vi "CreateSequence_Main.vi"(0 "Project Path":path, 5 "Measurement Name":string, 11 "error in (no error)":errorcluster) -> (15 "Error Out":errorcluster)   [LabVIEW 2021, in "Create Sequence.lvlib"]
uses:
  Create Sequence.lvlib
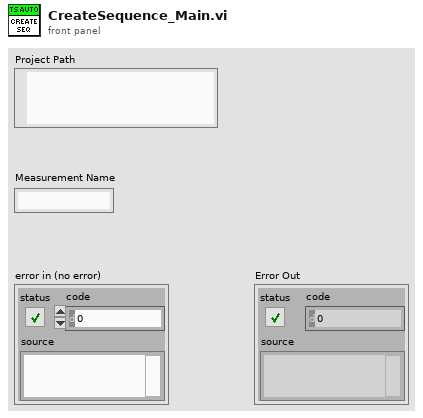
[diagram p1: front panel]
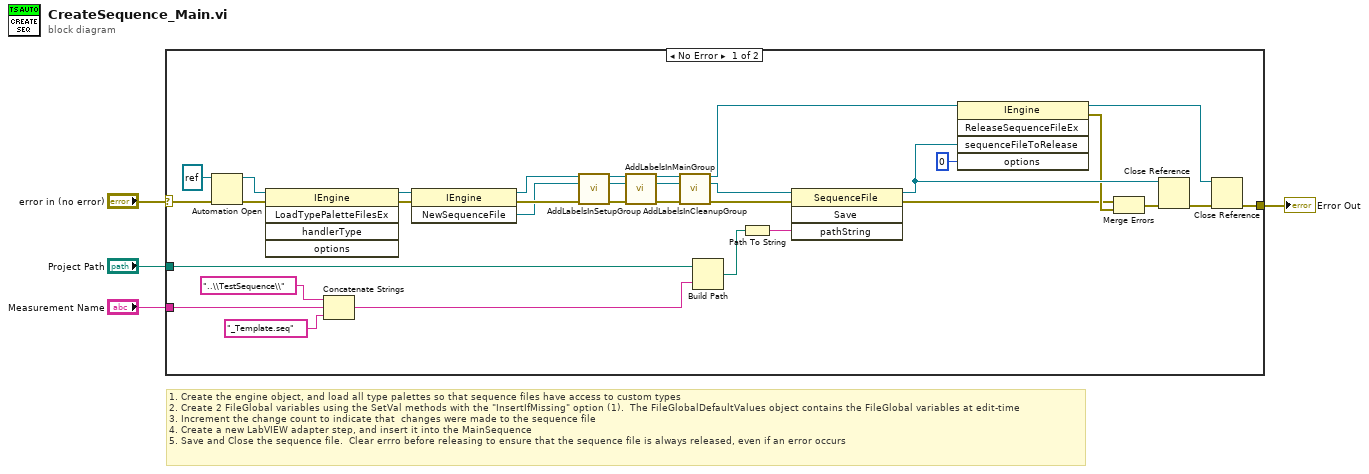
[diagram p0: block diagram]
diagram:
  # "1. Create the engine object, and load all type palettes so that sequence files have access to custom types\n2. Create 2 FileGlobal variables using the SetVal methods with the \"InsertIfMissing\" option (1).  The FileGlobalDefaultValues object contains the FileGlobal variables at edit-time\n3. Increment the change count to indicate that  changes were made to the sequence file\n4. Create a new LabVIEW adapter step, and insert it into the MainSequence\n5. Save and Close the sequence file.  Clear errro before releasing to ensure that the sequence file is always released, even if an error occurs"
  n1 = case shown="No Error" "error in (no error)" {
    selector: "error in (no error)" -> [w17 w38]
    tunnel: [w29 w38] -> w4
    tunnel: "Measurement Name" -> [w15 _]
    tunnel: "Project Path" -> [w5 _]
    frame No Error {
      n2 = Automation Open(error in (no error)=w17, Automation Refnum=refnum<k7> refnum) -> (Automation Refnum=w21:refnum<k7>, error out=w25:errorcluster)  [unwired: 2 in]
      n3 = invoke class="IEngine" method="LoadTypePaletteFilesEx"(reference=w21, error in=w25) -> (reference out=w26:refnum<k7>, error out=w24:errorcluster)  [unwired: 3 in, 3 out]
      n4 = Concatenate Strings("..\\TestSequence\\" ("string"), w15, "_Template.seq" ("string")) -> (w13:string)
      n5 = invoke class="IEngine" method="NewSequenceFile"(reference=w26, error in=w24) -> (reference out=w28:refnum<k7>, error out=w27:errorcluster, "NewSequenceFile"=w22:refnum<k7>)  [unwired: 1 in]
      n6 = call "AddLabelsInSetupGroup.vi"("Engine In"=w28, "SequenceFile In"=w22, "Error In"=w27) -> ("Engine Out"=w11:refnum<k7>, "SequenceFile Out"=w9:refnum<k7>, "Error Out"=w7:errorcluster)  [unwired: 10 in]
      n7 = call "AddLabelsInMainGroup.vi"("Engine In"=w11, "SequenceFile In"=w9, "Error In"=w7) -> ("Engine Out"=w12:refnum<k7>, "SequenceFile Out"=w10:refnum<k7>, "Error Out"=w8:errorcluster)  [unwired: 10 in]
      n8 = call "AddLabelsInCleanupGroup.vi"("Engine In"=w12, "SequenceFile In"=w10, "Error In"=w8) -> ("Engine Out"=w20:refnum<k7>, "SequenceFile Out"=w19:refnum<k7>, "Error Out"=w18:errorcluster)  [unwired: 10 in]
      n9 = Build Path(base path=w5, name or relative path=w13) -> (appended path=w30:path)
      n10 = Path To String(path=w30) -> (string=w36:string)
      n11 = invoke class="SequenceFile" method="Save"(reference=w19, error in=w18, "pathString"=w36) -> (reference out=w34:refnum<k7>, error out=w31:errorcluster)  [unwired: 1 in, 2 out]
      n12 = invoke class="IEngine" method="ReleaseSequenceFileEx"(reference=w20, "sequenceFileToRelease"=w34, "options"=0) -> (reference out=w35:refnum<k7>, error out=w33:errorcluster)  [unwired: 2 in, 3 out]
      n13 = Merge Errors(w31, w33) -> (w32:errorcluster)
      n14 = Close Reference(reference=w34, error in (no error)=w32) -> (error out=w37:errorcluster)
      n15 = Close Reference(reference=w35, error in (no error)=w37) -> (error out=w29:errorcluster)
    }
    frame Error {
    }
  }
  "Error Out" <- w4
